vi "Graph_PII_Controller_v00.vi"(8 "Integrator (-1)":cluster{"I Cavity":i32, "I2 Cavity":i32}, 9 "PII out (-1)":i16, 10 "Control Cavity":T1={"Lock"=FALSE, "Hold"=FALSE, "P Gain"=0, "P BS"=-5, "I Gain"=0, "I BS"=-10, "I2 G"=0, "I2 BS"=-26, "Scan Amp"=0, "Scan Off"=0, "Scan FS"=0, "SFS BS"=0, "I Max value"=10000, "I2 Max value"=10000, "Scope.Offset"=0, "Trigger Direction"=enum."either", "Scan-PII thresh"=0}, 11 "OPO A Error":i16) -> (0 "Integrator":cluster{"I Cavity":i32, "I2 Cavity":i32}, 1 "PII out":i16, 3 "I too high?":bool)   [LabVIEW 2010]
doc: "This is a PII Controller used here to lock cavities. Pound-Drever-Hall error signals are fed in and the PII output is fed out. Designed by Seiji Armstrong, based on a design by Ben Sparkes."
uses:
  Strict Type Defs/PII individual.ctl
panel:
  in  "Integrator (-1)":cluster{"I Cavity":i32, "I2 Cavity":i32}
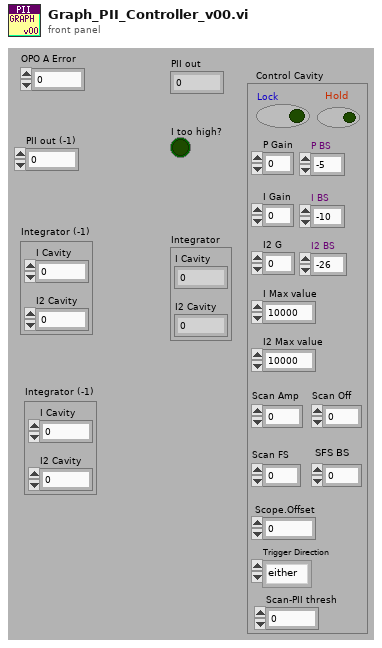
[diagram p1: front panel]
types:
  T1 = typedef "PII individual.ctl" = cluster{"Lock":bool, "Hold":bool, "P Gain":i32, "P BS":i16, "I Gain":i32, "I BS":i16, "I2 G":i32, "I2 BS":i16, "Scan Amp":i16, "Scan Off":i16, "Scan FS":u16, "SFS BS":i16, "I Max value":i32, "I2 Max value":i32, "Scope.Offset":i16, "Trigger Direction":enum8{"either", "minus-plus", "plus-minus"}, "Scan-PII thresh":i16}
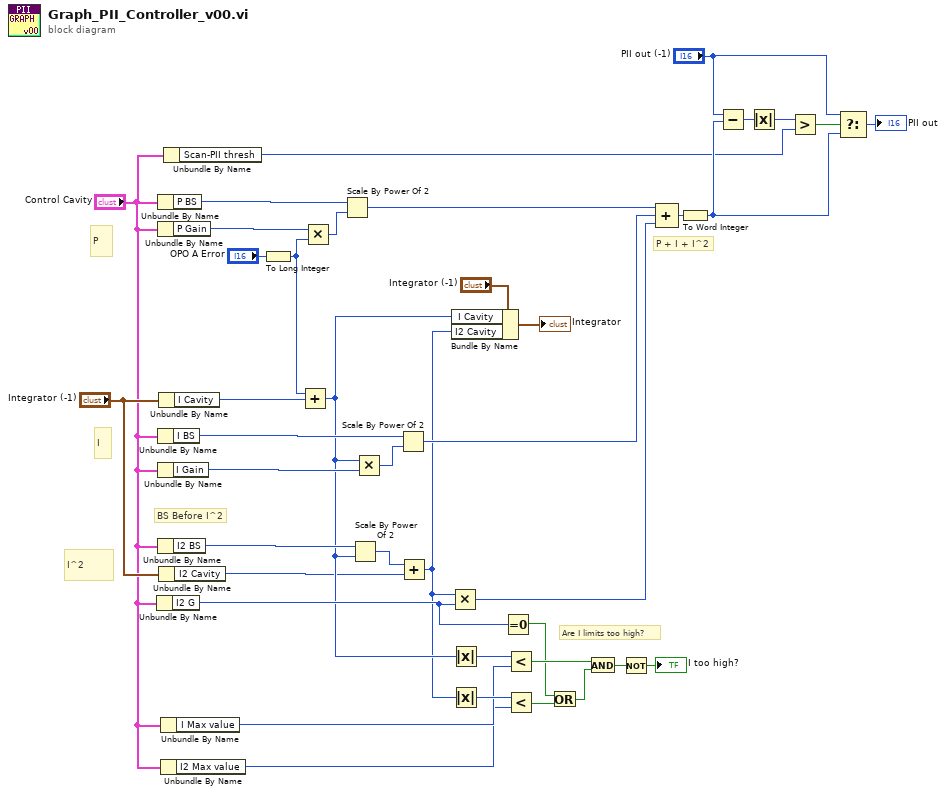
[diagram p0: block diagram]
diagram:
  # "I^2"
  # "Are I limits too high?"
  # "BS Before I^2"
  # "P"
  # "P + I + I^2"
  # "I"
  n1 = Unbundle By Name("Control Cavity") -> ("I2 G"=w28:i32)
  n2 = Unbundle By Name("Control Cavity") -> ("P BS"=w37:i16)
  n3 = Unbundle By Name("Control Cavity") -> ("P Gain"=w26:i32)
  n4 = Unbundle By Name("Control Cavity") -> ("I BS"=w35:i16)
  n5 = Unbundle By Name("Control Cavity") -> ("I Gain"=w36:i32)
  n6 = Unbundle By Name("Control Cavity") -> ("I2 BS"=w33:i16)
  n7 = Unbundle By Name("Integrator (-1)") -> ("I Cavity"=w16:i32)
  n8 = Unbundle By Name("Integrator (-1)") -> ("I2 Cavity"=w14:i32)
  n9 = Unbundle By Name("Control Cavity") -> ("I Max value"=w22:i32)
  n10 = Unbundle By Name("Control Cavity") -> ("I2 Max value"=w21:i32)
  n11 = Unbundle By Name("Control Cavity") -> ("Scan-PII thresh"=w1:i16)
  n12 = To Long Integer(number="OPO A Error") -> (32bit integer=w9:i32)
  n13 = Add(x=w9, y=w16) -> (x+y=w19:i32)
  n14 = Multiply(x=w26, y=w9) -> (x*y=w38:i32)
  n15 = Scale By Power Of 2(n=w37, x=w38) -> (x*2^n=w29:i32)
  n16 = Scale By Power Of 2(n=w33, x=w19) -> (x*2^n=w31:i32)
  n17 = Multiply(x=w19, y=w36) -> (x*y=w34:i32)
  n18 = Scale By Power Of 2(n=w35, x=w34) -> (x*2^n=w32:i32)
  n19 = Add(x=w31, y=w14) -> (x+y=w18:i32)
  n20 = Multiply(x=w18, y=w28) -> (x*y=w30:i32)
  n21 = Absolute Value(x=w19) -> (abs(x)=w40:i32)
  n22 = Absolute Value(x=w18) -> (abs(x)=w39:i32)
  n23 = Bundle By Name(cluster="Integrator (-1)", "I Cavity"=w19, "I2 Cavity"=w18) -> (→"Integrator":cluster{"I Cavity":i32, "I2 Cavity":i32})
  n24 = Equal To 0?(x=w28) -> (x = 0?=w11:bool)
  n25 = Less?(x=w40, y=w22) -> (x < y?=w25:bool)
  n26 = Less?(x=w39, y=w21) -> (x < y?=w12:bool)
  n27 = Or(x=w11, y=w12) -> (x .or. y?=w24:bool)
  n28 = And(x=w25, y=w24) -> (x .and. y?=w27:bool)
  n29 = Not(x=w27) -> (.not. x?=→"I too high?":bool)
  n30 = Compound Arithmetic op=ADD(w29, w32, w30) -> (w8:i32)
  n31 = To Word Integer(number=w8) -> (16bit integer=w5:i16)
  n32 = Subtract(x="PII out (-1)", y=w5) -> (x-y=w7:i16)
  n33 = Absolute Value(x=w7) -> (abs(x)=w2:i16)
  n34 = Greater?(x=w2, y=w1) -> (0:w6:bool)
  n35 = Select(t="PII out (-1)", s=w6, f=w5) -> (s? t:f=→"PII out":i16)
